vi "Anritsu VNA Set Learn String.vi"(7 "Anritsu VNA":T1, 8 "error in (no error)":errorcluster, 10 "Learn String":string, 11 "VISA Resource Name":refnum<visa-resource-name>) -> (0 "error out":errorcluster {"code" format="%.0x"}, 3 "dup VISA Resource Name":refnum<visa-resource-name>)   [LabVIEW 2011]
uses:
  TypeDefs/Anritsu VNA Instrument Info.ctl
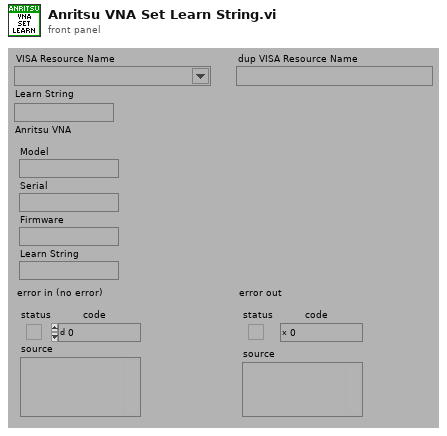
[diagram p1: front panel]
types:
  T1 = typedef "Anritsu VNA Instrument Info.ctl" = cluster{"Model":string, "Serial":string, "Firmware":string, "Learn String":string}
  T2 = typedef "Anritsu VNA Model.ctl" = enum16{"Not Supported", "37XXXX", "MS20XXX", "MS462XX", "MS464XX"}
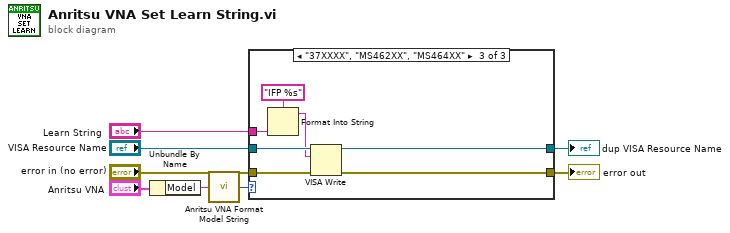
[diagram p0: block diagram]
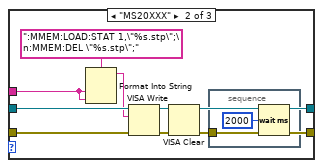
[diagram p3: hidden frame]
diagram:
  n1 = Unbundle By Name("Anritsu VNA") -> ("Model"=w2:string)
  n2 = call "Anritsu VNA Format Model String.vi"("Model"=w2) -> ("Model"=w1:T2)
  n3 = case shown="\"37XXXX\", \"MS462XX\", \"MS464XX\"" w1 {
    tunnel: [w9 w11 w22] -> w8
    tunnel: "error in (no error)" -> [w9 w19 w27]
    tunnel: "Learn String" -> [_ w15 w23]
    tunnel: "VISA Resource Name" -> [w10 w18 w26]
    tunnel: [w10 w12 w21] -> w4
    frame "Not Supported" {
    }
    frame "MS20XXX" {
      n4 = Format Into String(format string=":MMEM:LOAD:STAT 1,\"%s.stp\";\n:MMEM:DEL \"%s.stp\";", w15, w15) -> (resulting string=w16:string)  [unwired: 2 in, 1 out]
      n5 = VISA Write(VISA resource name=w18, write buffer=w16, error in (no error)=w19) -> (VISA resource name out=w13:refnum<visa-resource-name>, error out=w14:errorcluster)  [unwired: 1 out]
      n6 = VISA Clear(VISA resource name=w13, error in (no error)=w14) -> (VISA resource name out=w12:refnum<visa-resource-name>, error out=w11:errorcluster)
      n7 = stacked-sequence {
        tunnel: w11 -> [_]
        frame #0 {
          n8 = Wait (ms)(milliseconds to wait=u32 2000) -> ()  [unwired: 1 out]
        }
      }
    }
    frame "37XXXX", "MS462XX", "MS464XX" {
      n9 = Format Into String(format string="IFP %s", w23) -> (resulting string=w24:string)  [unwired: 2 in, 1 out]
      n10 = VISA Write(VISA resource name=w26, write buffer=w24, error in (no error)=w27) -> (VISA resource name out=w21:refnum<visa-resource-name>, error out=w22:errorcluster)  [unwired: 1 out]
    }
  }
  "error out" <- w8
  "dup VISA Resource Name" <- w4
